vi "get channel handle base value.vi"(8 "error in (no error)":errorcluster, 11 "device type":T1=enum."LAN") -> (0 "error out":errorcluster, 3 "channel handle base value":u16 format="%x")   [LabVIEW 2024, in "atsj peakcan basic.lvlib"]
doc: "Gets the <b>channel handle base value</b> associated with the specified <b>device type</b> / bus type."
uses:
  atsj peakcan basic.lvlib
  device type.ctl
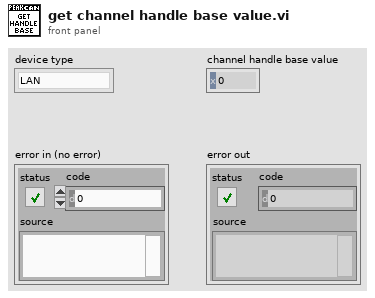
[diagram p1: front panel]
types:
  T1 = typedef "atsj peakcan basic.lvlib/device type.ctl" = enum8{"ISA", "DNG", "PCI", "USB", "PCC", "LAN"}
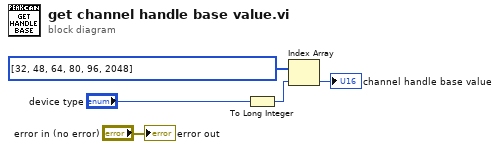
[diagram p0: block diagram]
diagram:
  n1 = To Long Integer(number="device type") -> (32bit integer=w4:i32)
  n2 = Index Array(array=u16[] [32, 48, 64, 80, 96, 2048] ("Array"), index=w4) -> (element=→"channel handle base value":u16)
  "error out" <- "error in (no error)"
